vi "transmisor PSK.vi"() -> ()   [LabVIEW 2016]
uses:
  <vilib>/addons/Modulation/Digital/Support/Controls/Pack Bits Parameters.ctl
  <vilib>/addons/Modulation/Analog/support/mod_Set Error Source.vi
  <vilib>/addons/Modulation/Digital/Support/Common/Validators/mod_Generate Filter Coefficients Validate.vi
  <vilib>/addons/Modulation/Digital/General/subVIs/mod_Generate Filter Coefficients.vi
  <vilib>/addons/Modulation/Digital/General/MT Generate PSK System Parameters(M).vi
  <instrlib>/niUSRP/niUSRP Write Tx Data (CDB Cluster).vi
  <vilib>/addons/Modulation/niDMT.lvlib
panel:
  out "session handle out":refnum<k15>
  in  "device names":refnum<k15>
  out "input bit stream":i8[](array[numeric])
  out "Frame Size [samples]":i32=4092
  out "Constellation Graph":T1(graph) caption="Tx Signal Constellation"
  in  "filter parameters":T2={"Alpha"=0.5, "Filter Length"=6, "TX Filter"=enum."Root Raised Cos"} {"Alpha" format="%.2f"}
  out "symbols out":cdb[](array[numeric]) format="%.2f"
  out "Symbol Rate\n[symbols/sec]":dbl=500000.0 format="%#.6p"
  in  "BIt":i32=10 format="%b"
  in  "stop":bool
  in  "Tx Parameters":T3={"Tx IQ Sampling\nRate [s/sec]"=400000.0, "Tx Frequency [Hz]"=915000000.0, "Tx Gain [dB]"=0.0, "Tx Antenna"="TX1"} {"Tx Gain [dB]" format="%#.6p"; "Tx Frequency [Hz]" format="%#.6p"; "Tx IQ Sampling\nRate [s/sec]" format="%#.6p"}
  out "Actual Tx Parameters":T3={"Tx IQ Sampling\nRate [s/sec]"=400000.0, "Tx Frequency [Hz]"=915000000.0, "Tx Gain [dB]"=0.0, "Tx Antenna"="TX1"} {"Tx Gain [dB]" format="%#.6p"; "Tx Frequency [Hz]" format="%#.6p"; "Tx IQ Sampling\nRate [s/sec]" format="%#.6p"}
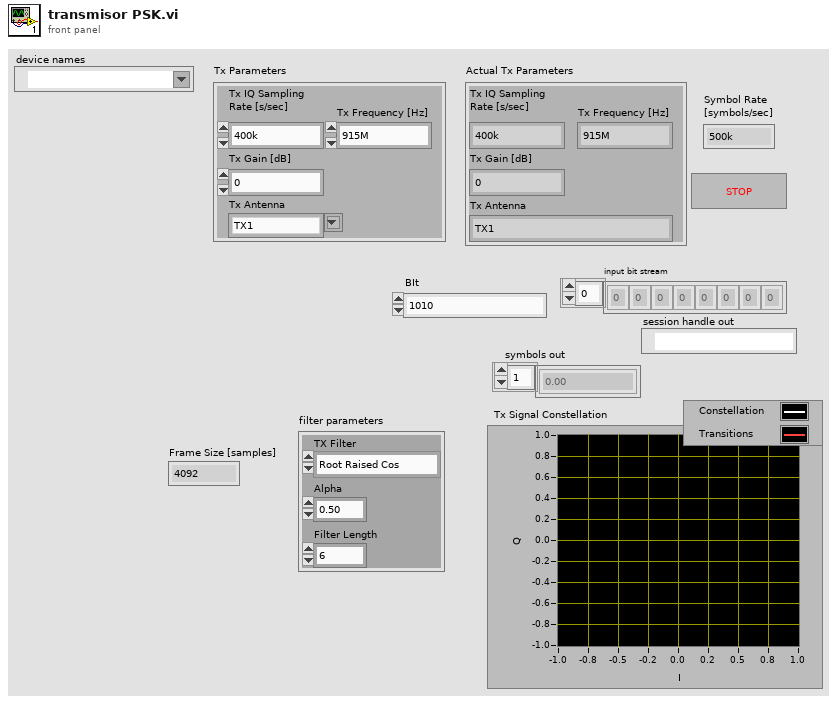
[diagram p1: front panel]
types:
  T1 = cluster{"constellation":dbl[], "oversampled data":dbl[]}[]
  T2 = cluster{"Alpha":dbl, "Filter Length":i32, "TX Filter":enum16{"none", "Raised Cosine", "Root Raised Cos", "Gaussian"}}
  T3 = cluster{"Tx IQ Sampling\nRate [s/sec]":dbl, "Tx Frequency [Hz]":dbl, "Tx Gain [dB]":dbl, "Tx Antenna":string}
  T4 = typedef "niDMT.lvlib/Pack Bits Parameters.ctl" = enum16{"Unsigned", "Signed"}
  T5 = enum16{"FSK", "PSK", "QAM", "MSK", "PAM", "ASK", "CPM"}
  T6 = enum16{"none", "Raised Cosine", "Root Raised Cos", "Gaussian"}
  T7 = cluster{"samples per symbol (16)":i32, "symbol map":cdb[], "differential PSK":enum16{"disable", "enable"}, "PSK type":u16}
  T8 = typedef "niAMT.lvlib/Complex Data Waveform.ctl" = cluster{"t0":dbl, "dt":dbl, "Y":cdb[]}
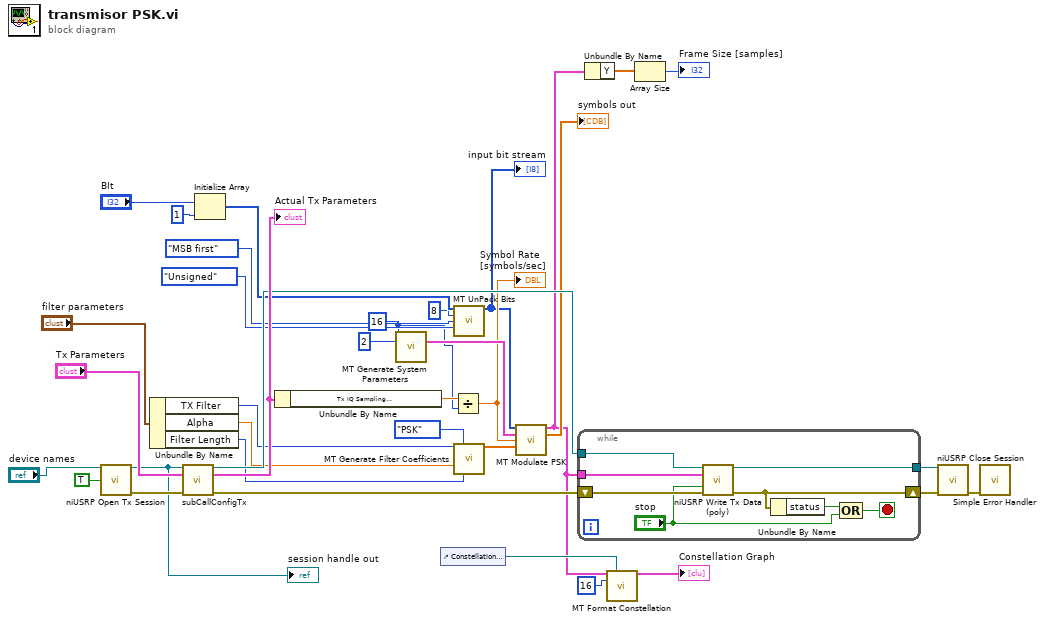
[diagram p0: block diagram]
diagram:
  w3 = 16 ("samples per symbol (16)")
  n1 = call <instrlib>:"niUSRP Open Tx Session.vi"("device names"="device names", "reset"=TRUE) -> ("session handle out"=w1:refnum<k15>, "error out"=w34:errorcluster)  [unwired: 12 in]
  "session handle out" <- w1
  n2 = Unbundle By Name("filter parameters") -> ("TX Filter"=w18:T6, "Alpha"=w17:dbl, "Filter Length"=w16:i32)
  n3 = call "subCallConfigTx.vi"("session handle"=w1, "Tx Parameters"="Tx Parameters", "error in"=w34) -> ("session handle out"=w29:refnum<k15>, "Actual Tx Parameters"=w35:T3, "error out"=w28:errorcluster)  [unwired: 10 in]
  "Actual Tx Parameters" <- w35
  n4 = Initialize Array("BIt", 1 ("dimension size")) -> (w8:i32[])
  n5 = Unbundle By Name(w35) -> ("Tx IQ Sampling\nRate [s/sec]"=w24:dbl)
  n6 = call-poly <vilib>:"MT Generate System Parameters.vi"("samples per symbol (16)"=w3, "M-PSK (4)"=2) -> ("PSK system parameters"=w26:T7)  [unwired: 11 in, 2 out]
  n7 = control-ref of="Constellation Graph"() -> (w15:refnum<vi>)
  n8 = Divide(x=w24, y=w3) -> (x/y=w23:dbl)
  "Symbol Rate\n[symbols/sec]" <- w23
  n9 = call <vilib>:"MT UnPack Bits.vi"("input integers"=w8, "bits per integer"=8, "packed bit order"=enum16{"MSB first", "LSB first"}."MSB first", "integer format"=Pack_Bits_Parameters."Unsigned") -> ("output bit stream"=w4:i8[])  [unwired: 10 in, 1 out]
  "input bit stream" <- w4
  n10 = call <vilib>:"MT Generate Filter Coefficients.vi"("pulse shaping filter (none)"=w18, "modulation type"=T5."PSK", "filter parameter"=w17, "filter length (symbols)"=w16) -> ("pulse shaping filter coefficients"=w21:dbl[])  [unwired: 9 in, 2 out]
  n11 = call <vilib>:"MT Modulate PSK.vi"("input bit stream"=w4, "PSK system parameters"=w26, "symbol rate (Hz)"=w23, "pulse shaping filter coefficients"=w21) -> ("output complex waveform"=w11:T8, "symbols out"=→"symbols out":cdb[])  [unwired: 9 in, 1 out]
  n12 = while {
    tunnel: [w42] -> w31
    tunnel: w29 -> [w44]
    shift-right: [w38] -> w32
    shift-left: w28 -> [w43]
    tunnel: w11 -> [w37]
    stop <- w41 stop-if-true
    n13 = call-poly <instrlib>:"niUSRP Write Tx Data (poly).vi"("session handle"=w44, "data"=w37, "end of data?"="stop", "error in (no error)"=w43) -> ("session handle out"=w42:refnum<k15>, "error out"=w38:errorcluster)  [unwired: 10 in]
    n14 = Unbundle By Name(w38) -> ("status"=w40:bool)
    n15 = Compound Arithmetic op=OR(w40, "stop") -> (w41:bool)
  }
  n16 = Unbundle By Name(w11) -> ("Y"=w10:cdb[])
  n17 = call <vilib>:"MT Format Constellation.vi"("waveform"=w11, "constellation reference"=w15, "samples per symbol"=16) -> ("constellation graph"=→"Constellation Graph":T1)  [unwired: 11 in, 1 out]
  n18 = Array Size(array=w10) -> (size(s)=→"Frame Size [samples]":i32)
  n19 = call <instrlib>:"niUSRP Close Session.vi"("session handle"=w31, "error in (no error)"=w32) -> ("error out"=w30:errorcluster)  [unwired: 13 in]
  n20 = call <vilib>:"Simple Error Handler.vi"("error in (no error)"=w30) -> ()  [unwired: 4 in, 5 out]
